vi "퀴즈.vi"() -> ()   [LabVIEW 2020]
uses:
  <vilib>/numeric/Random Number (Range) DBL.vi
panel:
  out "예제2_주사위 분석":dbl[](array[numeric])
  out "난수20개":dbl[](array[numeric])
  out "예제1_배열10":i32[](array[numeric])
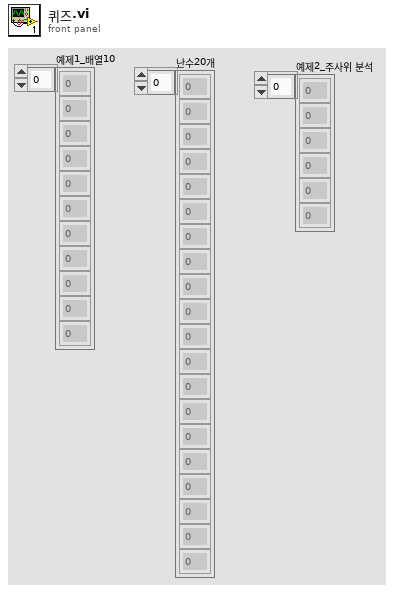
[diagram p1: front panel]
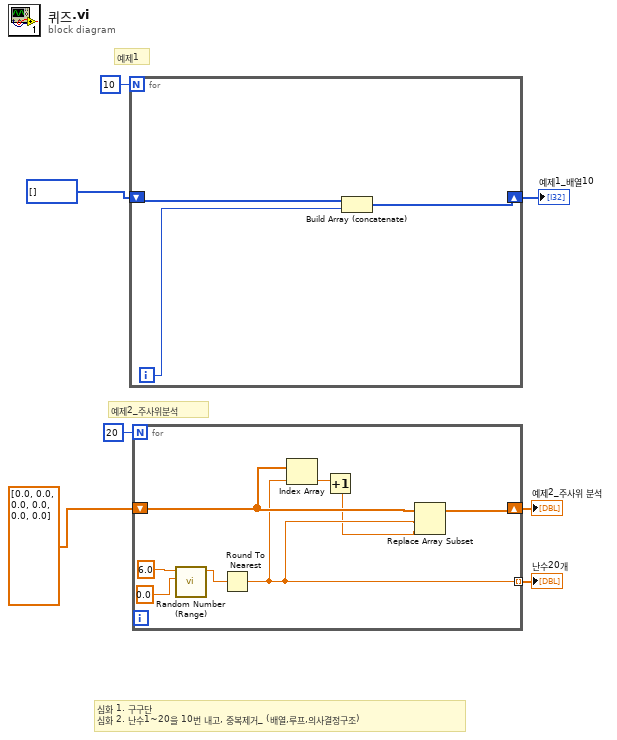
[diagram p0: block diagram]
diagram:
  # "심화 1. 구구단\n심화 2. 난수1~20을 10번 내고, 중복제거_ (배열,루프,의사결정구조)"
  # "예제2_주사위분석"
  # "예제1"
  n1 = for {
    N: 10 -> [_]
    shift-right: [w10] -> w6
    shift-left: i32[] [] -> [w9]
    i -> [w8]
    n2 = Build Array (concatenate)(w9, w8) -> (w10:i32[])
  }
  "예제1_배열10" <- w6
  n3 = for {
    N: 20 -> [_]
    shift-right: [w11] -> w1
    shift-left: dbl[] [0.0, 0.0, 0.0, 0.0, 0.0, 0.0] -> [w14]
    tunnel: [w13] -> w3 mode=indexing
    n4 = call-poly <vilib>:"Random Number (Range).vi"("lower bound (0)"=0.0, "upper bound (100)"=6.0 ("x/y")) -> ("number"=w16:dbl)  [unwired: 9 in]
    n5 = Round To Nearest(number=w16) -> (nearest integer value=w13:dbl)
    n6 = Index Array(array=w14, index=w13) -> (element=w15:dbl)
    n7 = Increment(x=w15) -> (x+1=w12:dbl)
    n8 = Replace Array Subset(array=w14, new element=w12, index=w13) -> (w11:dbl[])
  }
  "난수20개" <- w3
  "예제2_주사위 분석" <- w1
